vi "clear Complex Data.vi"(4 "error in (no error)":errorcluster, 7 "Complex Data":refnum<class "Complex Data.lvclass">) -> (0 "error out":errorcluster)   [LabVIEW 2017]
doc: "Destroys a Complex Data object and frees its allocated memory."
uses:
  C:/Program Files/Thorlabs/SpectralRadar/LabVIEW/2012/user.lib/SpectralRadar.llb/Complex Data.lvclass
  SpectralRadar.dll
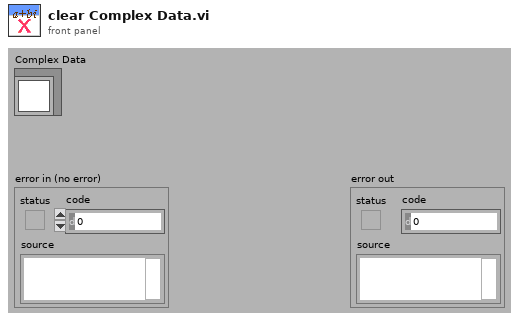
[diagram p1: front panel]
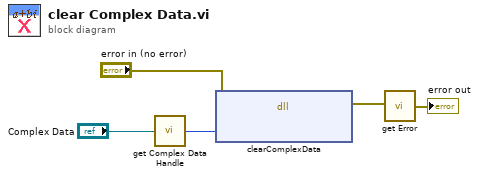
[diagram p0: block diagram]
diagram:
  n1 = call "get Complex Data Handle.vi"("Complex Data"="Complex Data") -> ("Handle"=w4:u64)
  n2 = dll-call lib="SpectralRadar.dll" fn="clearComplexData"(error in="error in (no error)", "Complex Data Handle"=w4) -> (error out=w3:errorcluster)  [unwired: 4 in, 1 out]
  n3 = call "get Error.vi"("error in (no error)"=w3) -> ("error out"=→"error out":errorcluster)
